vi "Rename Msg.vi"() -> ()   [LabVIEW 2021, in "_Refactor Msg.lvlib"]
uses:
  _Refactor Msg.lvlib
  <vilib>/Utility/EditLVLibs/Edit LVLibs.lvlib
panel:
  in  "Rename":bool
  in  "New Name":string
  in  "Message To Rename":path
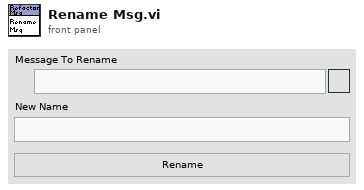
[diagram p1: front panel]
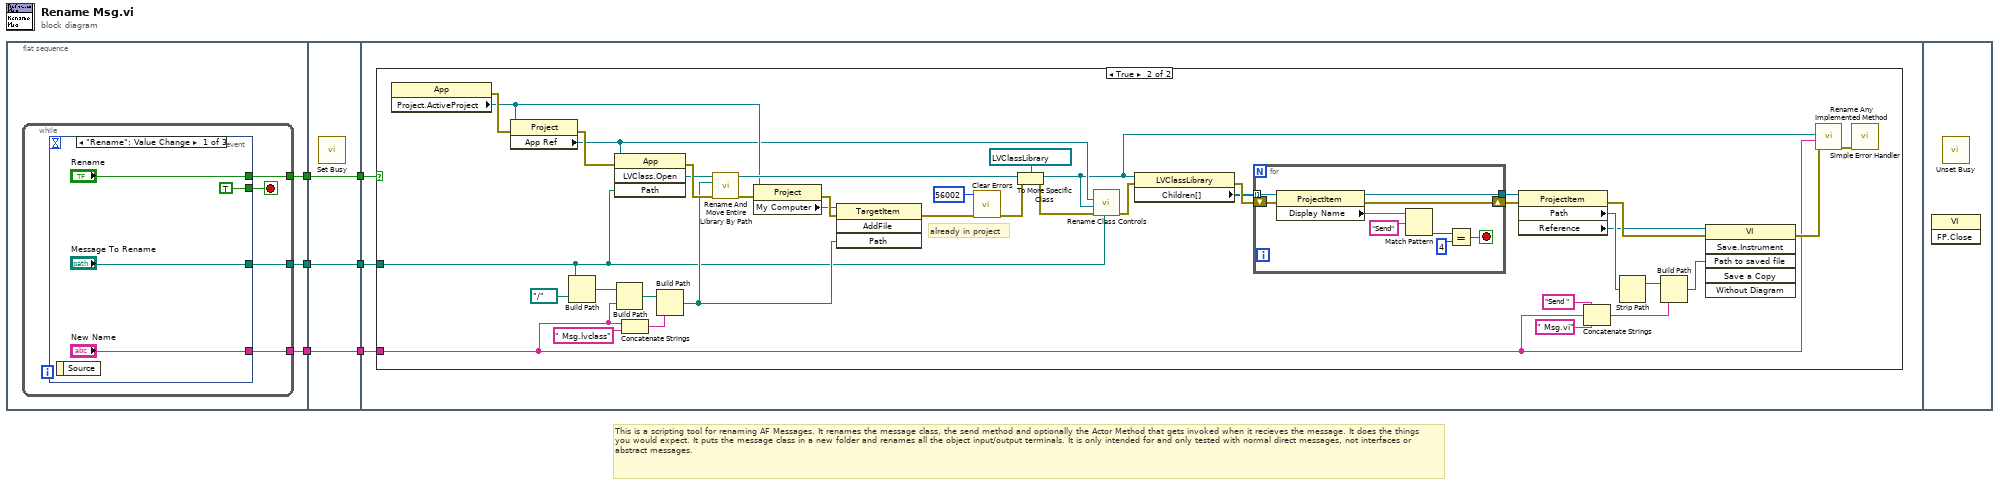
[diagram p0: block diagram]
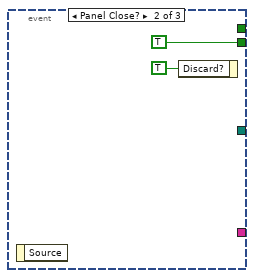
[diagram p2: hidden frame]
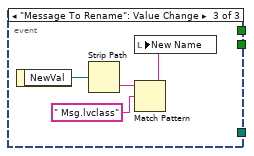
[diagram p3: hidden frame]
diagram:
  # "This is a scripting tool for renaming AF Messages. It renames the message class, the send method and optionally the Actor Method that gets invoked when it recieves the message. It does the things you would expect. It puts the message class in a new folder and renames all the object input/output terminals. It is only intended for and only tested with normal direct messages, not interfaces or abstract messages."
  n1 = flat-sequence {
    tunnel: [w9] -> w6
    tunnel: [w8] -> w5
    tunnel: [w7] -> w4
    tunnel: w6 -> [w26]
    tunnel: w5 -> [w25]
    tunnel: w4 -> [w24]
    tunnel: [w26] -> w3
    tunnel: [w25] -> w2
    tunnel: [w24] -> w1
    tunnel: w3 -> [w29]
    tunnel: w2 -> [w27]
    tunnel: w1 -> [w28]
    frame #0 {
      n2 = while {
        tunnel: [w13] -> w9
        tunnel: [w12] -> w8
        tunnel: [w11] -> w7
        stop <- w10 stop-if-true
        n3 = event shown="[0] \"Rename\": Value Change" {
          selector: _ -> [_ _ _]
          dyn-events: _ -> [_ _ _]
          timeout: _ -> [_ _ _]
          tunnel: ["Rename" _ _] -> w13
          tunnel: ["New Name" _ _] -> w12
          tunnel: ["Message To Rename" _ _] -> w11
          tunnel: [TRUE TRUE _] -> w10
          event "Rename": Value Change {
            n4 = event-data() -> ()  [unwired: 1 in, 1 out]
          }
          event Panel Close? {
            n5 = event-data() -> ()  [unwired: 1 in, 1 out]
            n6 = event-data("Discard?"=TRUE) -> ()  [unwired: 1 in, 1 out]
          }
          event "Message To Rename": Value Change {
            n7 = event-data() -> ("NewVal"=w23:path)  [unwired: 1 in]
            n8 = Strip Path(path=w23) -> (name=w22:string)  [unwired: 1 out]
            n9 = Match Pattern(string=w22, regular expression=" Msg.lvclass") -> (before substring=w20:string)  [unwired: 1 in, 3 out]
            n10 = local write "New Name"(w20) -> ()
          }
        }
      }
    }
    frame #1 {
      n11 = call <vilib>:"Set Busy.vi"() -> ()  [unwired: 10 in, 2 out]
    }
    frame #2 {
      n12 = case shown="True" w29 {
        tunnel: w28 -> [_ w35]
        tunnel: w27 -> [_ w30]
        frame False {
        }
        frame True {
          # "already in project"
          n13 = property class="App"() -> (error out=w62:errorcluster, "Project.ActiveProject"=w37:refnum<vi>)  [unwired: 2 in, 1 out]
          n14 = property class="Project"(reference=w37, error in=w62) -> (error out=w58:errorcluster, "App Ref"=w34:refnum<vi>)  [unwired: 1 out]
          n15 = Build Path(base path=w35, name or relative path=path "../..") -> (appended path=w55:path)
          n16 = invoke class="App" method="LVClass.Open"(reference=w34, error in=w58, "Path"=w35) -> (error out=w61:errorcluster, "LVClass.Open"=w57:refnum<vi>)  [unwired: 1 in, 2 out]
          n17 = Build Path(base path=w55, name or relative path=w30) -> (appended path=w54:path)
          n18 = Concatenate Strings(w30, " Msg.lvclass" ("string")) -> (w53:string)
          n19 = Build Path(base path=w54, name or relative path=w53) -> (appended path=w51:path)
          n20 = call <vilib>:"Rename And Move Entire Library By Path.vi"("error in (no error)"=w61, "New library path"=w51, "Library ref in"=w57) -> ("error out"=w36:errorcluster, "Library ref out"=w39:refnum<vi>)  [unwired: 7 in]
          n21 = property class="Project"(reference=w37, error in=w36) -> (error out=w68:errorcluster, "My Computer"=w38:refnum<vi>)  [unwired: 1 out]
          n22 = invoke class="TargetItem" method="AddFile"(reference=w38, error in=w68, "Path"=w51) -> (error out=w63:errorcluster)  [unwired: 1 in, 3 out]
          n23 = call <vilib>:"Clear Errors.vi"("error in (no error)"=w63, "specific error code to clear (0: all)"=56002) -> ("error out"=w60:errorcluster)  [unwired: 4 in, 1 out]
          n24 = To More Specific Class(target class=refnum<vi> refnum ("Class in"), reference=w39, error in=w60) -> (specific class reference=w31:refnum<vi>, error out=w59:errorcluster)
          n25 = call "Rename Class Controls.vi"("Old Class"=w35, "error in"=w59, "Class to Rename"=w31, "App Ref"=w34) -> ("error out"=w67:errorcluster)  [unwired: 7 in]
          n26 = property class="LVClassLibrary"(reference=w31, error in=w67) -> (error out=w66:errorcluster, "Children[]"=w50:refnum<vi>[])  [unwired: 1 out]
          n27 = for {
            tunnel: w50 -> [w75] mode=indexing
            shift-right: [w76] -> w65
            shift-left: w66 -> [w77]
            tunnel: [w73] -> w49
            stop <- w71 stop-if-true
            n28 = property class="ProjectItem"(reference=w75, error in=w77) -> (reference out=w73:refnum<vi>, error out=w76:errorcluster, "Display Name"=w72:string)
            n29 = Match Pattern(string=w72, regular expression="Send") -> (offset past match=w69:i32)  [unwired: 1 in, 3 out]
            n30 = Equal?(x=w69, y=4 ("x")) -> (x = y?=w71:bool)
          }
          n31 = property class="ProjectItem"(reference=w49, error in=w65) -> (error out=w64:errorcluster, "Path"=w48:path, "Reference"=w46:refnum<vi>)  [unwired: 1 out]
          n32 = Concatenate Strings("Send " ("string"), w30, " Msg.vi" ("string")) -> (w43:string)
          n33 = Strip Path(path=w48) -> (stripped path=w47:path)  [unwired: 1 out]
          n34 = Build Path(base path=w47, name or relative path=w43) -> (appended path=w42:path)
          n35 = invoke class="VI" method="Save.Instrument"(reference=w46, error in=w64, "Path to saved file"=w42) -> (error out=w32:errorcluster)  [unwired: 3 in, 5 out]
          n36 = call "Rename Any Implemented Method.vi"("error in"=w32, "Name"=w30, "Class To Rename"=w31) -> ("error out"=w33:errorcluster)  [unwired: 8 in]
          n37 = call <vilib>:"Simple Error Handler.vi"("error in (no error)"=w33) -> ()  [unwired: 4 in, 5 out]
        }
      }
    }
    frame #3 {
      n38 = invoke class="VI" method="FP.Close"() -> ()  [unwired: 3 in, 3 out]
      n39 = call <vilib>:"Unset Busy.vi"() -> ()  [unwired: 11 in, 1 out]
    }
  }
